vi "Register Sessions.vi"(8 "error in":errorcluster, 11 "session reservation in":refnum<class "Session Reservation.lvclass">) -> (0 "error out":errorcluster, 3 "session reservation out":refnum<class "Session Reservation.lvclass">)   [LabVIEW 2021, in "NI Session Management V1 Client.lvlib" / "Session Reservation.lvclass"]
doc: "Registers sessions with the session management service for shared use."
uses:
  Session Reservation.lvclass
  Session Reservation.lvclass/Session Reservation.ctl
  gRPC/Generated APIs/ni/measurementlink/sessionmanagement/v1/RPC Messages/ni_measurementlink_sessionmanagement_v1_RegisterSessionsRequest.ctl
  gRPC/Generated APIs/ni/measurementlink/sessionmanagement/v1/RPC Messages/ni_measurementlink_sessionmanagement_v1_SessionInformation.ctl
  gRPC/Generated APIs/ni/measurementlink/sessionmanagement/v1/RPC Messages/nidevice_grpc_Session.ctl
  gRPC/Generated APIs/ni/measurementlink/sessionmanagement/v1/RPC Messages/ni_measurementlink_sessionmanagement_v1_ChannelMapping.ctl
  gRPC/Generated APIs/ni/measurementlink/sessionmanagement/v1/RPC Messages/ni_measurementlink_sessionmanagement_v1_SessionInformation_AnnotationsEntry.ctl
  Measurements/Helpers/Error Strings Global Internal.vi
  <vilib>/Utility/error.llb/Error Cluster From Error Code.vi
  gRPC/Generated APIs/ni/measurementlink/sessionmanagement/v1/ni.measurementlink.sessionmanagement.v1.api.lvlib
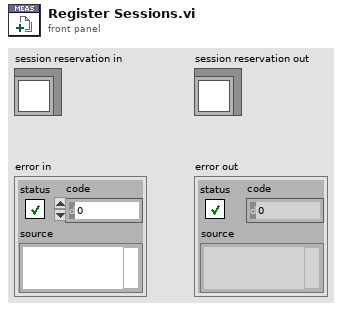
[diagram p1: front panel]
types:
  T1 = typedef "ni.measurementlink.sessionmanagement.v1.api.lvlib/ni_measurementlink_sessionmanagement_v1_RegisterSessionsRequest.ctl" = cluster{"sessions":T2[]}
  T2 = typedef "ni.measurementlink.sessionmanagement.v1.api.lvlib/ni_measurementlink_sessionmanagement_v1_SessionInformation.ctl" = cluster{"session":T3, "resource_name":string, "channel_list":string, "instrument_type_id":string, "session_exists":bool, "session_reserved":bool, "channel_mappings":T4[], "annotations":T5[]}
  T3 = typedef "ni.measurementlink.sessionmanagement.v1.api.lvlib/nidevice_grpc_Session.ctl" = cluster{"name":string}
  T4 = typedef "ni.measurementlink.sessionmanagement.v1.api.lvlib/ni_measurementlink_sessionmanagement_v1_ChannelMapping.ctl" = cluster{"pin_or_relay_name":string, "site":i32, "channel":string, "multiplexer_resource_name":string, "multiplexer_route":string}
  T5 = typedef "ni.measurementlink.sessionmanagement.v1.api.lvlib/ni_measurementlink_sessionmanagement_v1_SessionInformation_AnnotationsEntry.ctl" = cluster{"key":string, "value":string}
  T6 = typedef "NI Session Management V1 Client.lvlib/Session Reservation.lvclass/Data.ctl" = cluster{"session and driver infos":T7[], "pin or relay names":string[], "connection map":refnum<class "Connection Map.lvclass">, "pin map context":T9, "reservation observer":refnum<class "IReservation Observer.lvclass">, "dvr valid":bool, "group mappings":T10}
  T7 = typedef "NI Session Management V1 Client.lvlib/Session Reservation.lvclass/Session and Driver Info.ctl" = cluster{"session info":T2, "session":variant, "session factory":refnum<class "ISession Factory.lvclass">, "initialize and close session behavior":T8}
  T8 = typedef "NI Session Management Instrument.lvlib/ISession Factory.lvclass/Initialize and Close Session Behavior.ctl" = enum16{"Initialize and Close", "Attach and Detach", "Initialize and Detach", "Attach and Close"}
  T9 = typedef "ni.measurementlink.sessionmanagement.v1.api.lvlib/ni_measurementlink_PinMapContext.ctl" = cluster{"pin_map_id":string, "sites":i32[]}
  T10 = typedef "NI Session Management V1 Client.lvlib/Session Reservation.lvclass/Group Mapping.ctl" = map{string, string[]}
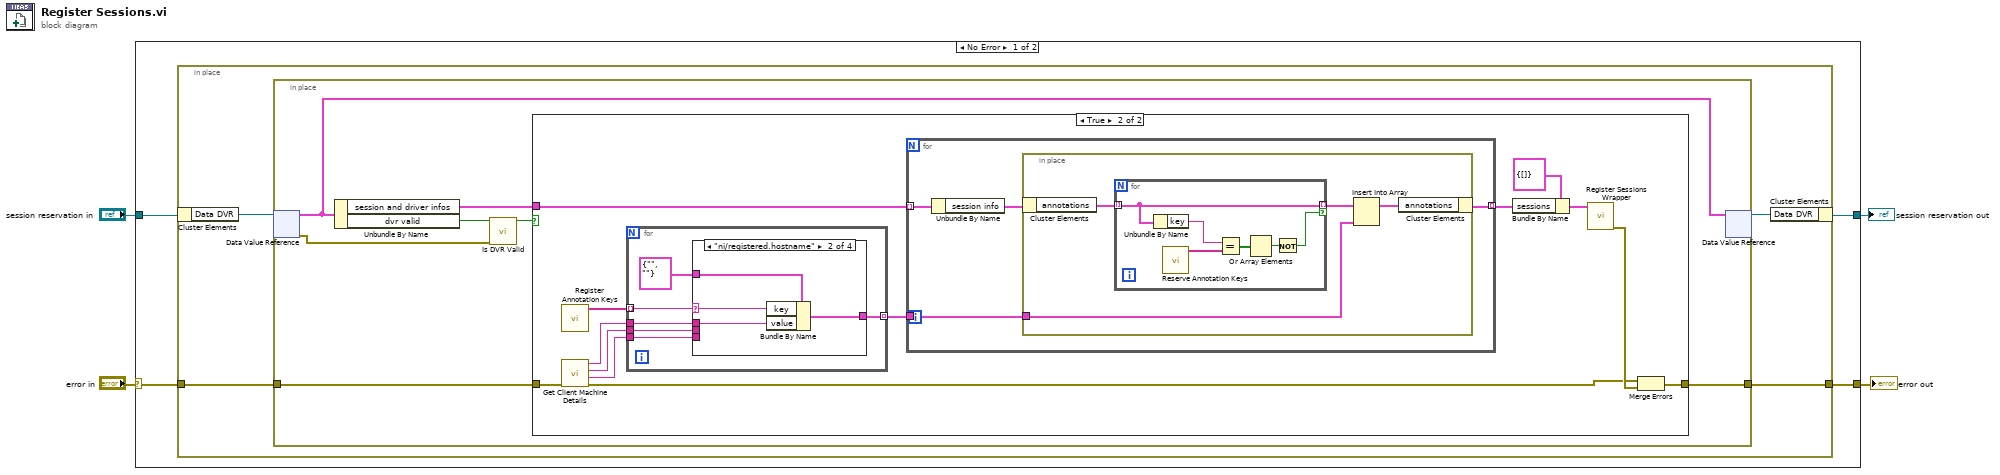
[diagram p0: block diagram]
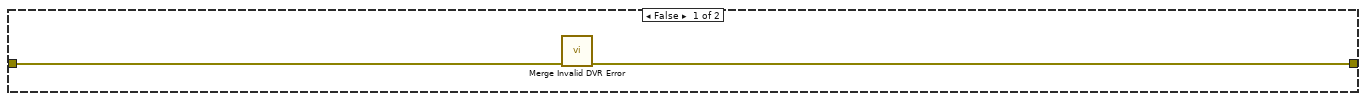
[diagram p2: hidden frame]
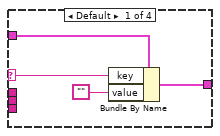
[diagram p3: hidden frame]
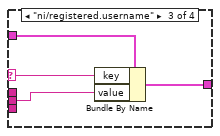
[diagram p4: hidden frame]
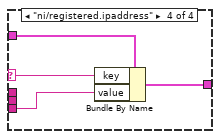
[diagram p5: hidden frame]
diagram:
  n1 = case shown="No Error" "error in" {
    selector: "error in" -> [w6 w71]
    tunnel: [w7 w72] -> w2
    tunnel: "session reservation in" -> [w8 w72]
    tunnel: [w5 w71] -> w1
    frame No Error {
      n2 = in-place {
        in-place-border: w6 -> [w10]
        in-place-border: [w9] -> w5
        n3 = in-place-cluster #1(w8) -> ("Data DVR"=w12:refnum<data-value>)
        n4 = in-place {
          in-place-border: w10 -> [w15]
          in-place-border: [w14] -> w9
          n5 = in-place-dvr #2(w12) -> (w13:T6, w18:errorcluster)
          n6 = Unbundle By Name(w13) -> ("session and driver infos"=w16:T7[], "dvr valid"=w19:bool)
          n7 = call "Is DVR Valid.vi"("dvr error in"=w18, "dvr valid in"=w19) -> ("dvr valid out"=w17:bool)  [unwired: 9 in]
          n8 = case shown="True" w17 {
            tunnel: w16 -> [_ w22]
            tunnel: w15 -> [w21 w31]
            tunnel: [w20 w33] -> w14
            frame False {
              n9 = call "Merge Invalid DVR Error.vi"("error in"=w21) -> ("error out"=w20:errorcluster)  [unwired: 10 in]
            }
            frame True {
              n10 = call "Register Annotation Keys.vi"() -> ("register annotation keys"=w27:string[])  [unwired: 11 in]
              n11 = call "Get Client Machine Details.vi"("error in"=w31) -> ("error out"=w23:errorcluster, "ip address"=w24:string, "username"=w25:string, "hostname"=w26:string)  [unwired: 7 in]
              n12 = for {
                tunnel: [w53] -> w28 mode=indexing
                tunnel: w27 -> [w52] mode=indexing
                tunnel: w24 -> [w51]
                tunnel: w25 -> [w50]
                tunnel: w26 -> [w49]
                n13 = case shown="\"ni/registered.hostname\"" w52 {
                  selector: w52 -> [w56 w61 w65 w69]
                  tunnel: T5 {"key"="", "value"=""} ("ni_measurementlink_sessionmanagement_v1_SessionInformation_AnnotationsEntry") -> [w58 w62 w66 w70]
                  tunnel: [w57 w60 w64 w68] -> w53
                  tunnel: w51 -> [_ _ _ w67]
                  tunnel: w50 -> [_ _ w63 _]
                  tunnel: w49 -> [_ w59 _ _]
                  frame Default {
                    n14 = Bundle By Name(cluster=w58, "key"=w56, "value"="") -> (w57:T5)
                  }
                  frame "ni/registered.hostname" {
                    n15 = Bundle By Name(cluster=w62, "key"=w61, "value"=w59) -> (w60:T5)
                  }
                  frame "ni/registered.username" {
                    n16 = Bundle By Name(cluster=w66, "key"=w65, "value"=w63) -> (w64:T5)
                  }
                  frame "ni/registered.ipaddress" {
                    n17 = Bundle By Name(cluster=w70, "key"=w69, "value"=w67) -> (w68:T5)
                  }
                }
              }
              n18 = for {
                tunnel: w22 -> [w38] mode=indexing
                tunnel: [w36] -> w32 mode=indexing
                tunnel: w28 -> [w35]
                n19 = Unbundle By Name(w38) -> ("session info"=w37:T2)
                n20 = in-place {
                  in-place-border: w35 -> [w40]
                  n21 = in-place-cluster #3(w37) -> ("annotations"=w39:T5[])
                  n22 = for {
                    tunnel: [w45] -> w41 mode=indexing if=w46
                    tunnel: w39 -> [w45] mode=indexing
                    n23 = Unbundle By Name(w45) -> ("key"=w43:string)
                    n24 = call "Reserve Annotation Keys.vi"() -> ("reserve annotation keys"=w44:string[])  [unwired: 11 in]
                    n25 = Equal?(x=w43, y=w44) -> (x = y?=w47:bool[])
                    n26 = Or Array Elements(Boolean array=w47) -> (logical OR=w48:bool)
                    n27 = Not(x=w48) -> (.not. x?=w46:bool)
                  }
                  n28 = Insert Into Array(array=w41, new element=w40) -> (w42:T5[])  [unwired: 1 in]
                  n29 = in-place-cluster #3("annotations"=w42) -> (w36:T2)
                }
              }
              n30 = Bundle By Name(cluster=T1 {"sessions"=[]} ("Request Data"), "sessions"=w32) -> (w30:T1)
              n31 = call "Register Sessions Wrapper.vi"("request data"=w30) -> ("error out"=w29:errorcluster)  [unwired: 9 in, 1 out]
              n32 = Merge Errors(w23, w29) -> (w33:errorcluster)
            }
          }
          n33 = in-place-dvr #2(w13) -> (w11:refnum<data-value>)  [unwired: 1 out]
        }
        n34 = in-place-cluster #1("Data DVR"=w11) -> (w7:refnum<class "Session Reservation.lvclass">)
      }
    }
    frame Error {
    }
  }
  "error out" <- w1
  "session reservation out" <- w2
